vi "open reentrant instance.vi"(8 "error in":errorcluster, 11 "function":T1) -> (0 "error out":errorcluster, 3 "reentrant instance":T1)   [LabVIEW 2014, in "call function by reference.lvclass"]
uses:
  call function by reference.lvclass
  function definition.ctl
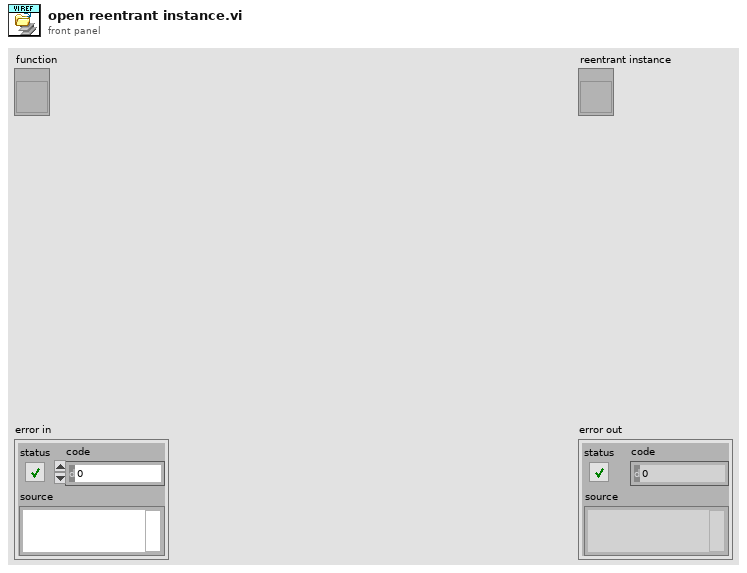
[diagram p1: front panel]
types:
  T1 = typedef "call function by reference.lvclass/function definition.ctl" = refnum<vi>
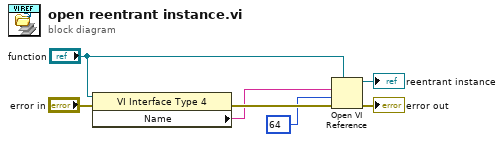
[diagram p0: block diagram]
diagram:
  n1 = property class="VI Interface Type 4"(reference="function", error in="error in") -> (error out=w6:errorcluster, "Name"=w2:string)  [unwired: 1 out]
  n2 = Open VI Reference(type specifier VI Refnum (for type only)="function", vi path=w2, options=64, error in (no error)=w6) -> (vi reference=→"reentrant instance":T1, error out=→"error out":errorcluster)  [unwired: 2 in]
